vi "start_delay_autocorrect_MD.vi"   [LabVIEW 2012]
uses:
  GFG/GFGnumericGet.vi
  GFG/GFGbooleanGet.vi
  GFG/GFGfpRefGet.vi
  GFG/GFGImageRefsGet.vi
  GFG/GFG library.lvlib
types:
  T1 = enum32{"Channel 1", "Channel 2", "Channel 3", "Channel 4", "Channel 5", "all channels", "RGB overlay", "ROI", "arbitrary line scan"}
  T2 = typedef "IMAQ Image.ctl" = refnum<image>
  T3 = cluster{"Channel 1 small":T2, "Channel 2 small":T2, "Channel 3 small":T2, "Channel 4 small":T2, "Channel 1 large":T2, "Channel 2 large":T2, "Channel 3 large":T2, "Channel 4 large":T2, "RGB overlay":T2, "ROI Image display":T2, "arb line scan display":T2, "Channel 5 large":T2}
  T4 = cluster{"WaveformChartRef":refnum<vi>, "DigitalRef":refnum<vi>, "ArrayRef":refnum<vi>, "TabControlRef":refnum<vi>, "EnumRef":refnum<vi>, "RingRef":refnum<vi>, "BooleanRef":refnum<vi>, "KnobRef":refnum<vi>, "SlideRef":refnum<vi>, "PathRef":refnum<vi>, "StringRef":refnum<vi>, "ComboBox":refnum<vi>, "WaveformGraphRef":refnum<vi>}
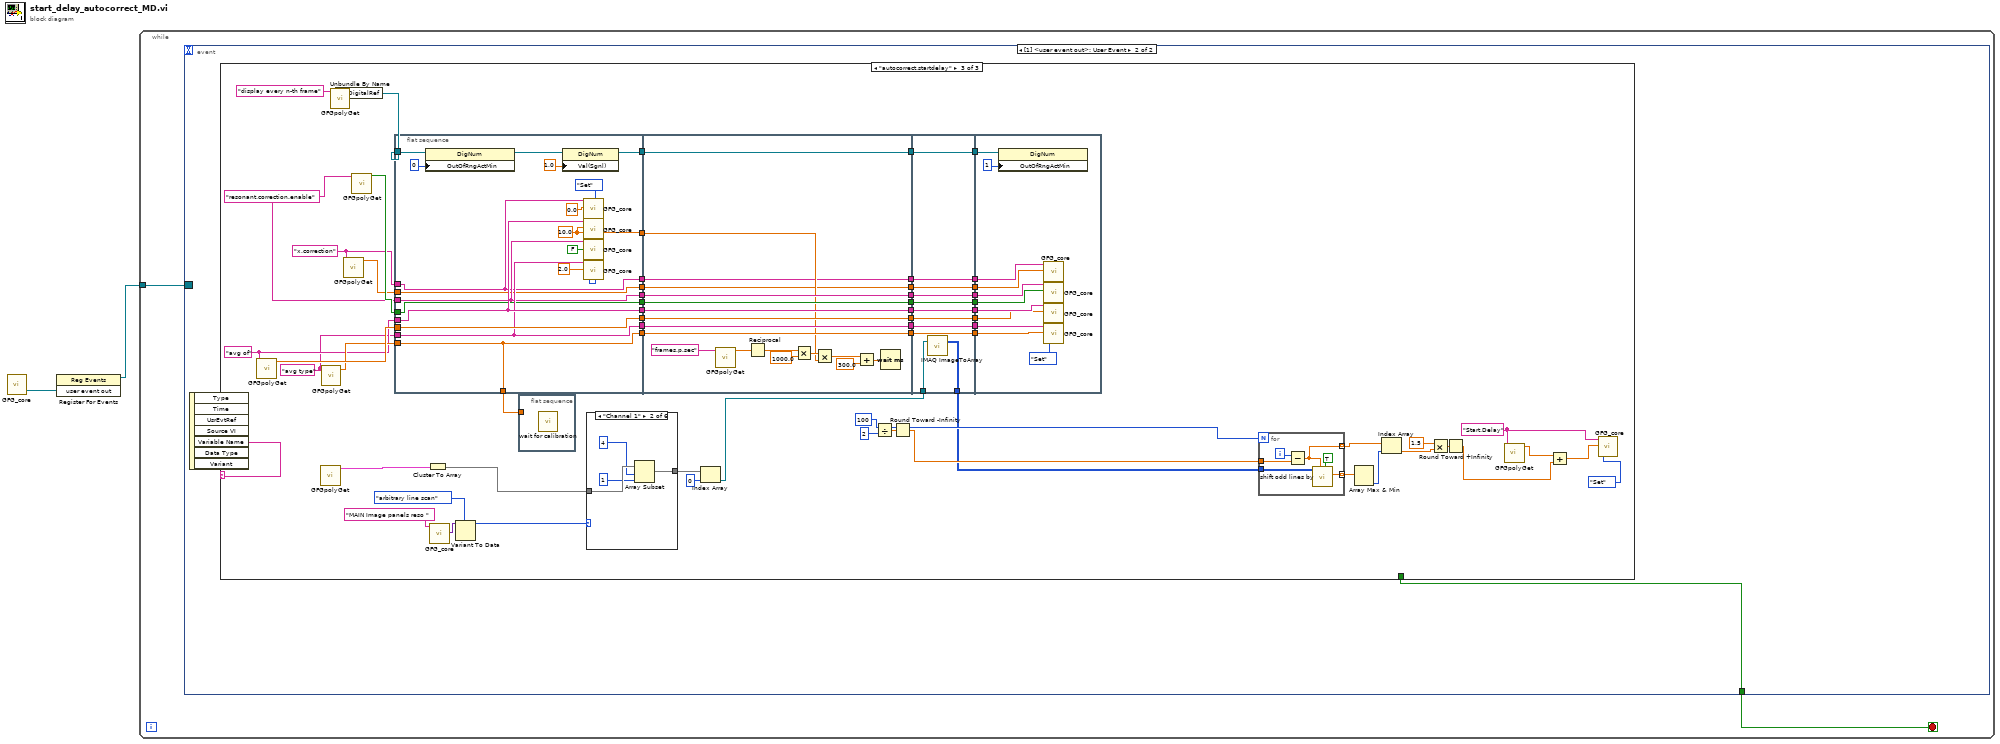
[diagram p0: block diagram]
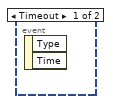
[diagram p2: hidden frame]
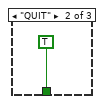
[diagram p4: hidden frame]
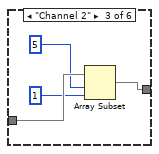
[diagram p6: hidden frame]
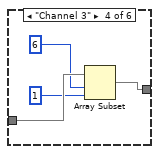
[diagram p7: hidden frame]
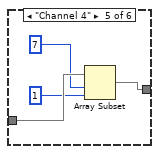
[diagram p8: hidden frame]
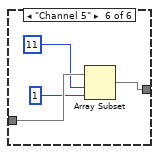
[diagram p9: hidden frame]
diagram:
  n1 = call "GFG_core.vi"() -> ("user event out"=w2:refnum<user-event>)  [unwired: 13 in, 6 out]
  n2 = register-events(w2) -> (reference out=w1:refnum<event-registration>)  [unwired: 2 in, 1 out]
  n3 = while {
    tunnel: w1 -> [w4]
    stop <- w3 stop-if-true
    n4 = event shown="[1] <user event out>: User Event" {
      selector: w4 -> [_ _]
      dyn-events: _ -> [_ _]
      timeout: _ -> [_ _]
      tunnel: [_ w5] -> w3
      event Timeout {
        n5 = event-data() -> ()  [unwired: 1 in, 2 out]
      }
      event User Event {
        n6 = event-data() -> ("Variable Name"=w6:string)  [unwired: 1 in, 6 out]
        n7 = case shown="\"autocorrect.startdelay\"" w6 {
          tunnel: [_ TRUE _] -> w5
          frame "False", Default {
          }
          frame "QUIT" {
          }
          frame "autocorrect.startdelay" {
            w14 = "x.correction" ("Variable Name in")
            w41 = "avg type" ("Variable Name in")
            w42 = "avg of" ("Variable Name in")
            w48 = "resonant.correction.enable" ("Variable Name in")
            w51 = "Start.Delay" ("Variable Name in")
            w72 = 100 ("Numeric")
            n8 = call-poly "GFGpolyGet.vi"("Variable Name in"=w42) -> ("Numeric"=w47:dbl)  [unwired: 9 in, 1 out]
            n9 = call-poly "GFGpolyGet.vi"() -> ("Image Refs Out"=w56:T3)  [unwired: 10 in, 1 out]
            n10 = call-poly "GFGpolyGet.vi"("Variable Name in"=w41) -> ("Numeric"=w46:dbl)  [unwired: 9 in, 1 out]
            n11 = call-poly "GFGpolyGet.vi"("Variable Name in"="display every n-th frame") -> ("output cluster"=w44:T4)  [unwired: 9 in, 1 out]
            n12 = Unbundle By Name(w44) -> ("DigitalRef"=w43:refnum<vi>)
            n13 = call-poly "GFGpolyGet.vi"("Variable Name in"=w14) -> ("Numeric"=w15:dbl)  [unwired: 9 in, 1 out]
            n14 = call-poly "GFGpolyGet.vi"("Variable Name in"=w48) -> ("Boolean"=w49:bool)  [unwired: 10 in]
            n15 = flat-sequence {
              tunnel: w49 -> [w79]
              tunnel: w48 -> [w80]
              tunnel: w47 -> [w82]
              tunnel: w46 -> [w77]
              tunnel: w43 -> [w90]
              tunnel: w42 -> [w83]
              tunnel: w41 -> [w81]
              tunnel: [w85] -> w32
              tunnel: [w83] -> w30
              tunnel: [w82] -> w28
              tunnel: [w81] -> w26
              tunnel: [w77] -> w24
              tunnel: [w80] -> w22
              tunnel: [w79] -> w20
              tunnel: [w78] -> w18
              tunnel: [w77] -> w16
              tunnel: w15 -> [w74]
              tunnel: w14 -> [w75]
              tunnel: [w75] -> w13
              tunnel: [w74] -> w8
              tunnel: w32 -> [w108]
              tunnel: [w108] -> w31
              tunnel: w30 -> [w107]
              tunnel: [w107] -> w29
              tunnel: w28 -> [w106]
              tunnel: [w106] -> w27
              tunnel: w26 -> [w105]
              tunnel: [w105] -> w25
              tunnel: w24 -> [w104]
              tunnel: [w104] -> w23
              tunnel: w22 -> [w103]
              tunnel: [w103] -> w21
              tunnel: w20 -> [w102]
              tunnel: [w102] -> w19
              tunnel: w18 -> [w96]
              tunnel: w13 -> [w92]
              tunnel: [w92] -> w12
              tunnel: [w91] -> w9
              tunnel: w8 -> [w91]
              tunnel: [w111] -> w40
              tunnel: [w119] -> w39
              tunnel: w31 -> [w119]
              tunnel: [w118] -> w38
              tunnel: w29 -> [w118]
              tunnel: [w117] -> w37
              tunnel: w27 -> [w117]
              tunnel: [w116] -> w36
              tunnel: w25 -> [w116]
              tunnel: [w115] -> w35
              tunnel: w23 -> [w115]
              tunnel: [w114] -> w34
              tunnel: w21 -> [w114]
              tunnel: [w113] -> w33
              tunnel: w19 -> [w113]
              tunnel: w17 -> [w112]
              tunnel: w12 -> [w110]
              tunnel: [w110] -> w11
              tunnel: [w109] -> w10
              tunnel: w9 -> [w109]
              tunnel: w39 -> [w129]
              tunnel: w38 -> [w128]
              tunnel: w37 -> [w127]
              tunnel: w36 -> [w126]
              tunnel: w35 -> [w125]
              tunnel: w34 -> [w124]
              tunnel: w33 -> [w123]
              tunnel: w11 -> [w122]
              tunnel: w10 -> [w121]
              frame #0 {
                w73 = enum16{"Init", "Set", "Get"}."Set" ("Action")
                w78 = 10.0 ("Numeric")
                n16 = property class="DigNum"(reference=w90, "OutOfRngActMin"=u8 0 ("Response to Value Outside Limits:Minimum")) -> (reference out=w88:refnum<vi>)  [unwired: 1 in, 1 out]
                n17 = property class="DigNum"(reference=w88, "Val(Sgnl)"=1.0 ("Numeric")) -> (reference out=w85:refnum<vi>)  [unwired: 1 in, 1 out]
                n18 = call "GFG_core.vi"("Variable Name in"=w75, "Variant in"=0.0 ("Numeric"), "Action"=w73) -> ()  [unwired: 10 in, 7 out]
                n19 = call "GFG_core.vi"("Variable Name in"=w83, "Variant in"=w78, "Action"=w73) -> ()  [unwired: 10 in, 7 out]
                n20 = call "GFG_core.vi"("Variable Name in"=w80, "Variant in"=FALSE ("Found/Replaced"), "Action"=w73) -> ()  [unwired: 10 in, 7 out]
                n21 = call "GFG_core.vi"("Variable Name in"=w81, "Variant in"=2.0 ("Numeric"), "Action"=w73) -> ()  [unwired: 10 in, 7 out]
              }
              frame #1 {
                n22 = call-poly "GFGpolyGet.vi"("Variable Name in"="frames.p.sec") -> ("Numeric"=w100:dbl)  [unwired: 9 in, 1 out]
                n23 = Reciprocal(x=w100) -> (1/x=w99:dbl)
                n24 = Multiply(x=w99, y=1000.0) -> (x*y=w97:dbl)
                n25 = Multiply(x=w97, y=w96) -> (x*y=w95:dbl)
                n26 = Add(x=w95, y=300.0) -> (x+y=w94:dbl)
                n27 = Wait (ms)(milliseconds to wait=w94) -> ()  [unwired: 1 out]
              }
              frame #2 {
                n28 = call "IMAQ ImageToArray"("Image"=w112) -> ("Image Pixels (I16)"=w111:i16[][])  [unwired: 3 in, 4 out]
              }
              frame #3 {
                w120 = enum16{"Init", "Set", "Get"}."Set" ("Action")
                n29 = property class="DigNum"(reference=w129, "OutOfRngActMin"=u8 1 ("Response to Value Outside Limits:Minimum")) -> ()  [unwired: 1 in, 2 out]
                n30 = call "GFG_core.vi"("Variable Name in"=w122, "Variant in"=w121, "Action"=w120) -> ()  [unwired: 10 in, 7 out]
                n31 = call "GFG_core.vi"("Variable Name in"=w124, "Variant in"=w123, "Action"=w120) -> ()  [unwired: 10 in, 7 out]
                n32 = call "GFG_core.vi"("Variable Name in"=w128, "Variant in"=w127, "Action"=w120) -> ()  [unwired: 10 in, 7 out]
                n33 = call "GFG_core.vi"("Variable Name in"=w126, "Variant in"=w125, "Action"=w120) -> ()  [unwired: 10 in, 7 out]
              }
            }
            n34 = Cluster To Array(cluster=w56) -> (array=w55:T2[])
            n35 = call "GFG_core.vi"("Variable Name in"="MAIN Image panels reso ") -> ("Variant Out"=w59:variant)  [unwired: 12 in, 6 out]
            n36 = Variant To Data(type=T1."arbitrary line scan" ("MAIN Image panels"), Variant=w59) -> (data=w57:T1)  [unwired: 1 in, 1 out]
            n37 = flat-sequence {
              tunnel: w16 -> [_]
              frame #0 {
                n38 = call "wait for calibration.vi"() -> ()  [unwired: 12 in]
              }
            }
            n39 = case shown="\"Channel 1\"" w57 {
              tunnel: w55 -> [_ w134 w138 w142 w146 w150]
              tunnel: [_ w131 w135 w139 w143 w147] -> w54
              frame Default {
              }
              frame "Channel 1" {
                n40 = Array Subset(array=w134, index=4, length=1) -> (w131:T2[])
              }
              frame "Channel 2" {
                n41 = Array Subset(array=w138, index=5, length=1) -> (w135:T2[])
              }
              frame "Channel 3" {
                n42 = Array Subset(array=w142, index=6, length=1 ("index")) -> (w139:T2[])
              }
              frame "Channel 4" {
                n43 = Array Subset(array=w146, index=7, length=1 ("index")) -> (w143:T2[])
              }
              frame "Channel 5" {
                n44 = Array Subset(array=w150, index=11, length=1 ("index")) -> (w147:T2[])
              }
            }
            n45 = Index Array(array=w54, index=0) -> (element=w17:T2)
            n46 = Divide(x=w72, y=2) -> (x/y=w70:dbl)
            n47 = Round Toward -Infinity(1:w70) -> (0:w69:dbl)
            n48 = for {
              N: w72 -> [_]
              tunnel: w40 -> [w156]
              tunnel: w69 -> [w155]
              tunnel: [w154] -> w68 mode=indexing
              tunnel: [w151] -> w66 mode=indexing
              i -> [w153]
              n49 = Subtract(x=w153, y=w155) -> (x-y=w151:dbl)
              n50 = call "shift odd lines by.vi"("calculate squared difference"=TRUE, "shift odd lines by"=w151, "frame in"=w156) -> ("squared difference"=w154:dbl)  [unwired: 7 in, 1 out]
            }
            n51 = Array Max & Min(array=w68) -> (min index (indices)=w67:i32)  [unwired: 3 out]
            n52 = Index Array(array=w66, index=w67) -> (element=w65:dbl)
            n53 = Multiply(x=1.5, y=w65) -> (x*y=w63:dbl)
            n54 = Round Toward +Infinity(x=w63) -> (ceil(x): smallest int >= x=w61:dbl)
            n55 = call-poly "GFGpolyGet.vi"("Variable Name in"=w51) -> ("Numeric"=w62:dbl)  [unwired: 9 in, 1 out]
            n56 = Add(x=w62, y=w61) -> (x+y=w50:dbl)
            n57 = call "GFG_core.vi"("Variable Name in"=w51, "Variant in"=w50, "Action"=enum16{"Init", "Set", "Get"}."Set") -> ()  [unwired: 10 in, 7 out]
          }
        }
      }
    }
  }
